vi "Open CiUsbLib.vi"(8 "error in (no error)":errorcluster, 11 "BMC in":refnum<class "BMC.lvclass">) -> (0 "error out":errorcluster, 2 "Automation Refnum":T1, 3 "BMC out":refnum<class "BMC.lvclass">)   [LabVIEW 2012, in "BMC.lvclass"]
uses:
  BMC.lvclass
  Controls/CIUsbKub.IHostDrv.ctl
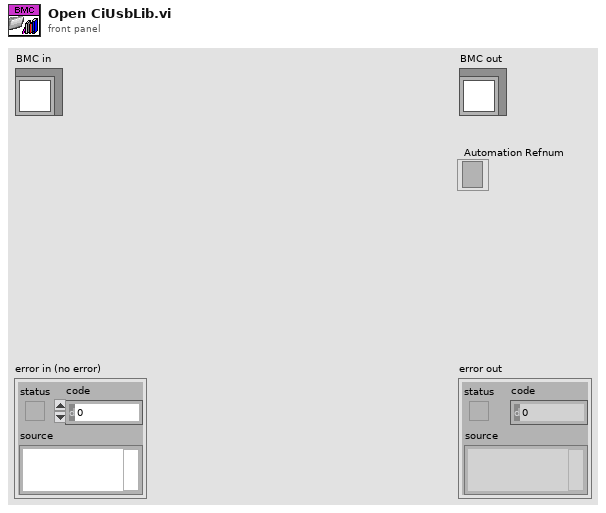
[diagram p1: front panel]
types:
  T1 = typedef "BMC.lvclass/CIUsbKub.IHostDrv.ctl" = refnum<k7>
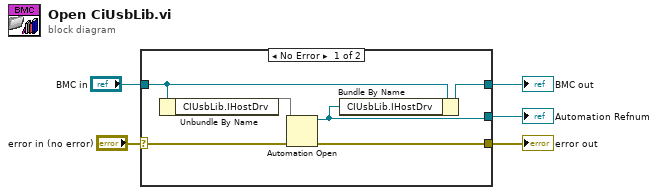
[diagram p0: block diagram]
diagram:
  n1 = case shown="No Error" "error in (no error)" {
    selector: "error in (no error)" -> [w11 w13]
    tunnel: [w7 w13] -> w4
    tunnel: [w10 w12] -> w2
    tunnel: "BMC in" -> [w9 w12]
    tunnel: [w6 _] -> w1
    frame No Error {
      n2 = Unbundle By Name(w9) -> ("CIUsbLib.IHostDrv"=w8)
      n3 = Automation Open(error in (no error)=w11, Automation Refnum=w8) -> (Automation Refnum=w6:T1, error out=w7:errorcluster)  [unwired: 2 out]
      n4 = Bundle By Name(cluster=w9, "CIUsbLib.IHostDrv"=w6) -> (w10:refnum<class "BMC.lvclass">)
    }
    frame Error {
    }
  }
  "error out" <- w4
  "BMC out" <- w2
  "Automation Refnum" <- w1
